vi "Processed_Bytes_To_RREQ_Packet.vi"(3 "error in (no error)":errorcluster, 4 "Processed Bytes":u8[](array[numeric]), 5 "RREQ Packet In":T2) -> (0 "error out":errorcluster, 1 "RREQ Param":T1, 2 "RREQ Packet Out":T2)   [LabVIEW 2017]
uses:
  Controls/Packet/Packet.ctl
  Controls/Packet/Packet_Direction.ctl
  Controls/Packet/Packet_Type.ctl
  Controls/Packet/Packet_Priority.ctl
  Controls/Control Packets/RREQ_Param.ctl
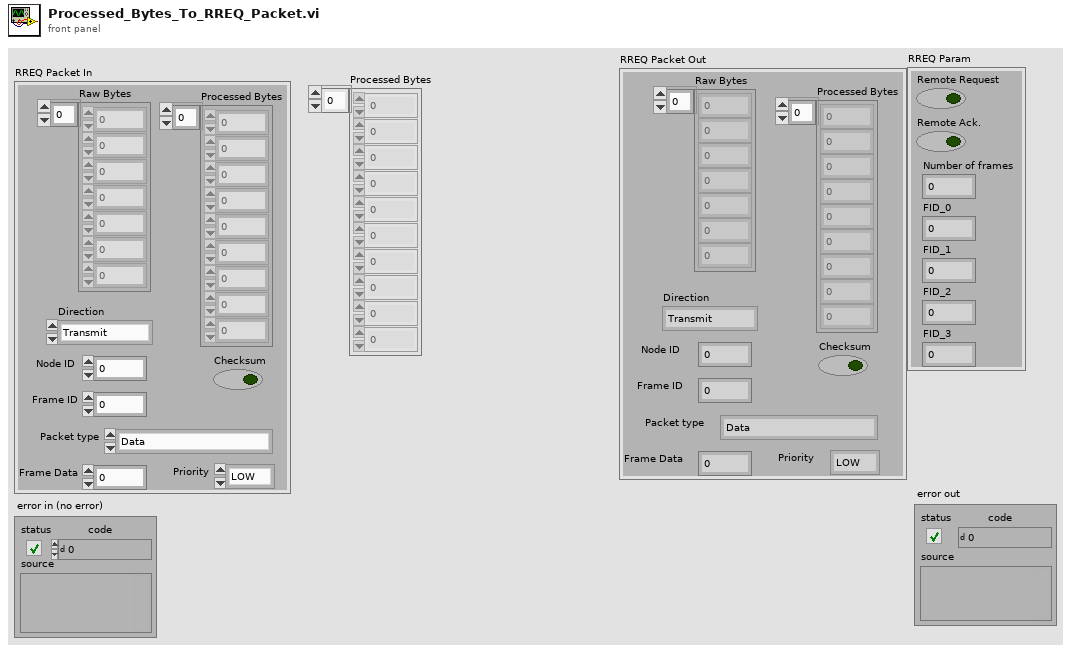
[diagram p1: front panel]
types:
  T1 = typedef "RREQ_Param.ctl" = cluster{"Remote Request":bool, "Remote Ack.":bool, "Number of frames":u8, "FID_0":u8, "FID_1":u8, "FID_2":u8, "FID_3":u8}
  T2 = typedef "Packet.ctl" = cluster{"Raw Bytes":u8[], "Checksum":bool, "Direction":T3, "Processed Bytes":u8[], "Node ID":u8, "Packet type":T4, "Frame Data":u32, "Priority":T5, "Frame ID":u8}
  T3 = typedef "Packet_Direction.ctl" = enum16{"Transmit", "Receive", "Bidirectional"}
  T4 = typedef "Packet_Type.ctl" = enum16{"Data", "Connection Management", "Remote Request", "Error/Status"}
  T5 = typedef "Packet_Priority.ctl" = enum16{"LOW", "HIGH"}
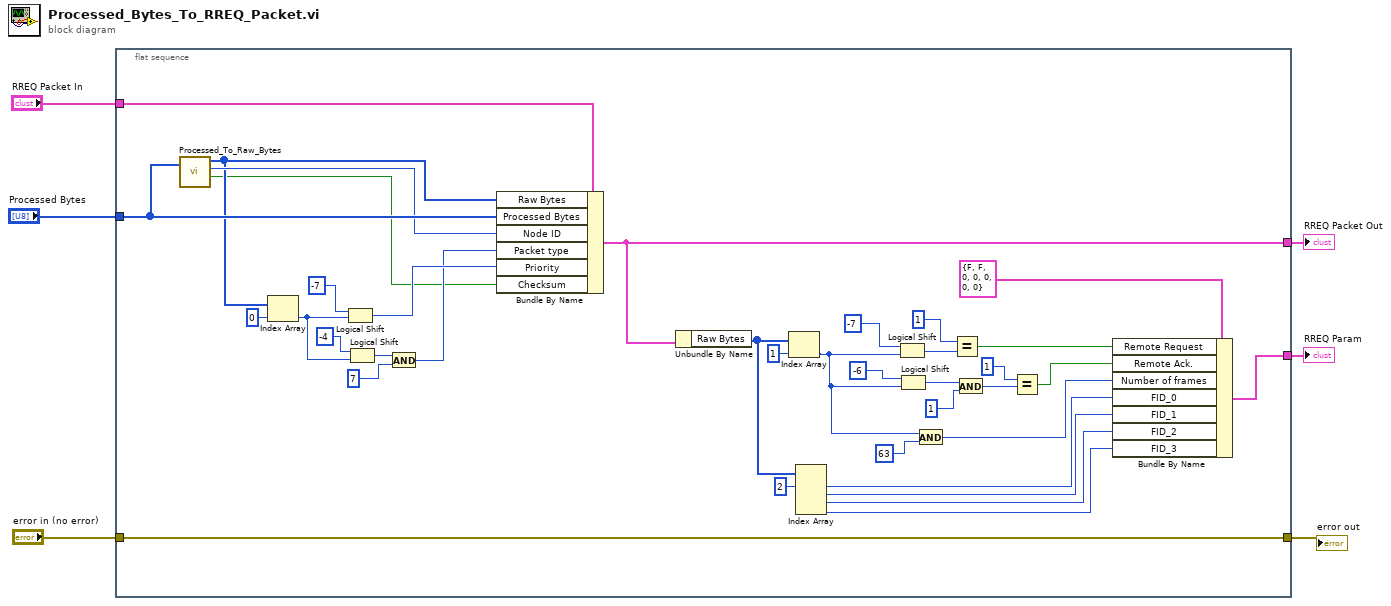
[diagram p0: block diagram]
diagram:
  n1 = flat-sequence {
    tunnel: "error in (no error)" -> [w43]
    tunnel: [w43] -> w1
    tunnel: "Processed Bytes" -> [w41]
    tunnel: "RREQ Packet In" -> [w42]
    tunnel: [w29] -> w3
    tunnel: [w13] -> w2
    frame #0 {
      n2 = call "Processed_To_Raw_Bytes.vi"("Processed Bytes"=w41) -> ("Checksum"=w30:bool, "Node ID"=w40:u8, "Raw Bytes"=w39:u8[])  [unwired: 1 in, 2 out]
      n3 = Index Array(array=w39, index=0) -> (element=w35:u8)
      n4 = Logical Shift(y=i16 -7, x=w35) -> (x << y=w36:u8)
      n5 = Logical Shift(y=i16 -4, x=w35) -> (x << y=w33:u8)
      n6 = And(x=w33, y=u8 7) -> (x .and. y?=w31:u8)
      n7 = Bundle By Name(cluster=w42, "Raw Bytes"=w39, "Processed Bytes"=w41, "Node ID"=w40, "Packet type"=w31, "Priority"=w36, "Checksum"=w30) -> (w29:T2)
      n8 = Unbundle By Name(w29) -> ("Raw Bytes"=w20:u8[])
      n9 = Index Array(array=w20, index=1) -> (element=w12:u8)
      n10 = Index Array(array=w20, index #1=2 ("index")) -> (element #1=w11:u8, element #2=w10:u8, element #3=w9:u8, element #4=w8:u8)  [unwired: 3 in]
      n11 = Logical Shift(y=i16 -7, x=w12) -> (x << y=w24:u8)
      n12 = Logical Shift(y=i16 -6, x=w12) -> (x << y=w25:u8)
      n13 = And(x=w12, y=u8 63) -> (x .and. y?=w7:u8)
      n14 = Equal?(x=u8 1, y=w24) -> (x = y?=w15:bool)
      n15 = And(x=w25, y=u8 1) -> (x .and. y?=w22:u8)
      n16 = Equal?(x=u8 1, y=w22) -> (x = y?=w14:bool)
      n17 = Bundle By Name(cluster=T1 {"Remote Request"=FALSE, "Remote Ack."=FALSE, "Number of frames"=0, "FID_0"=0, "FID_1"=0, "FID_2"=0, "FID_3"=0} ("Cluster"), "Remote Request"=w15, "Remote Ack."=w14, "Number of frames"=w7, "FID_0"=w11, "FID_1"=w10, "FID_2"=w9, "FID_3"=w8) -> (w13:T1)
    }
  }
  "RREQ Packet Out" <- w3
  "RREQ Param" <- w2
  "error out" <- w1
